vi "Add to Application MUXList.vi"(7 "Replace if found? (F)":bool, 8 "error in (no error)":errorcluster, 9 "Destinations":string[](array[string]), 10 "Source":string, 11 "SLSC Switch in":refnum<class "SLSC Switch.lvclass">) -> (0 "error out":errorcluster, 1 "New Entry?":bool, 3 "SLSC Switch out":refnum<class "SLSC Switch.lvclass">)   [LabVIEW 2016, in "SLSC Switch.lvlib" / "SLSC Switch.lvclass"]
uses:
  SLSC Switch.lvclass
  SLSC Switch.lvclass/SLSC Switch.ctl
  Controls/MuxList Entry.ctl
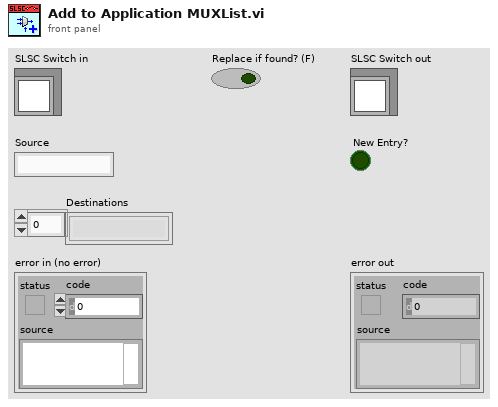
[diagram p1: front panel]
types:
  T1 = typedef "SLSC Switch.lvlib/SLSC Switch.lvclass/MuxList Entry.ctl" = cluster{"Source":string, "Destinations":string[]}
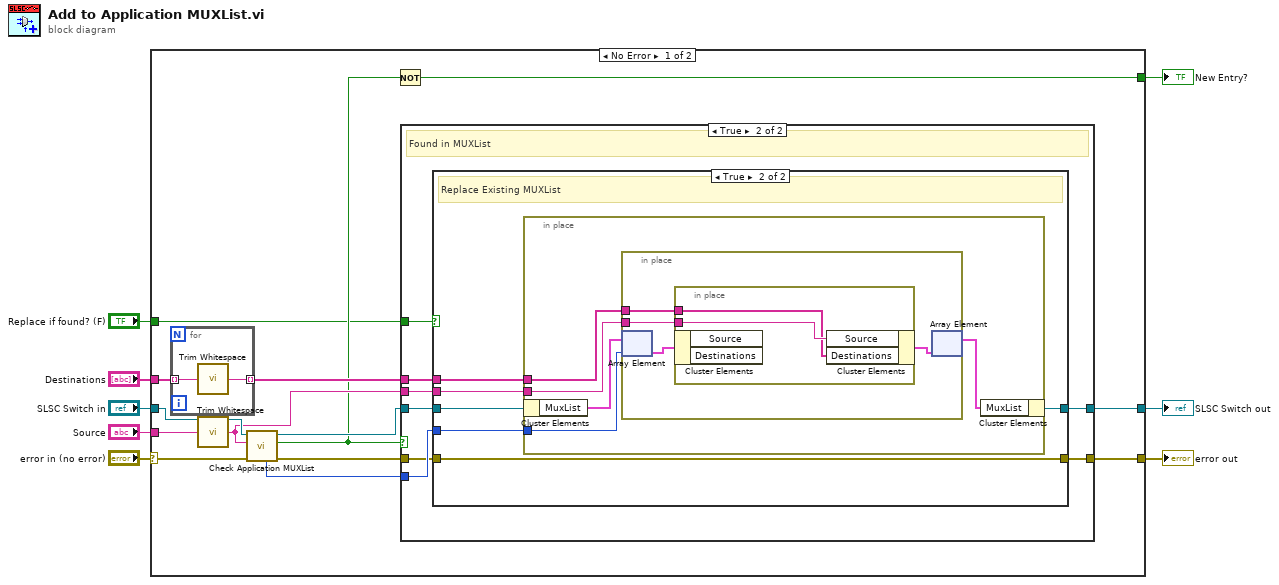
[diagram p0: block diagram]
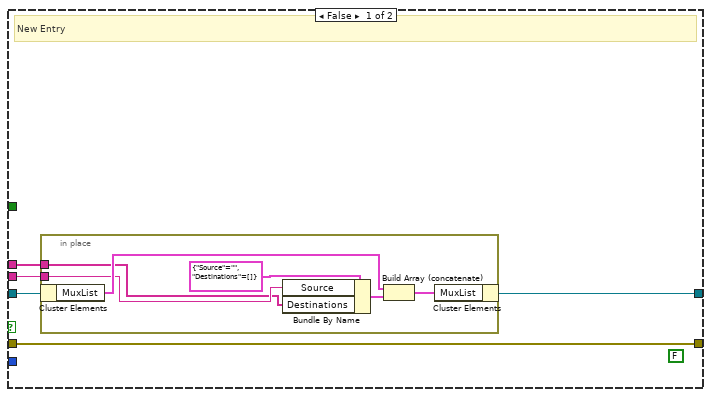
[diagram p2: hidden frame]
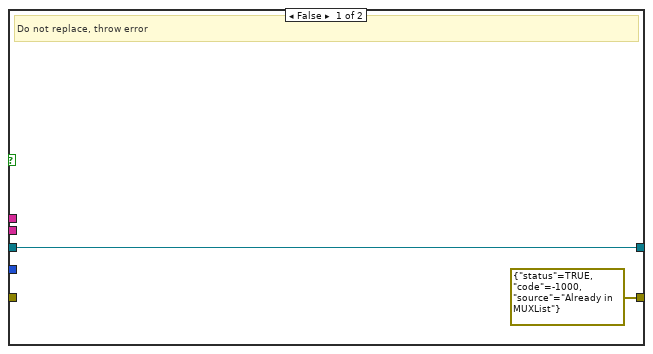
[diagram p3: hidden frame]
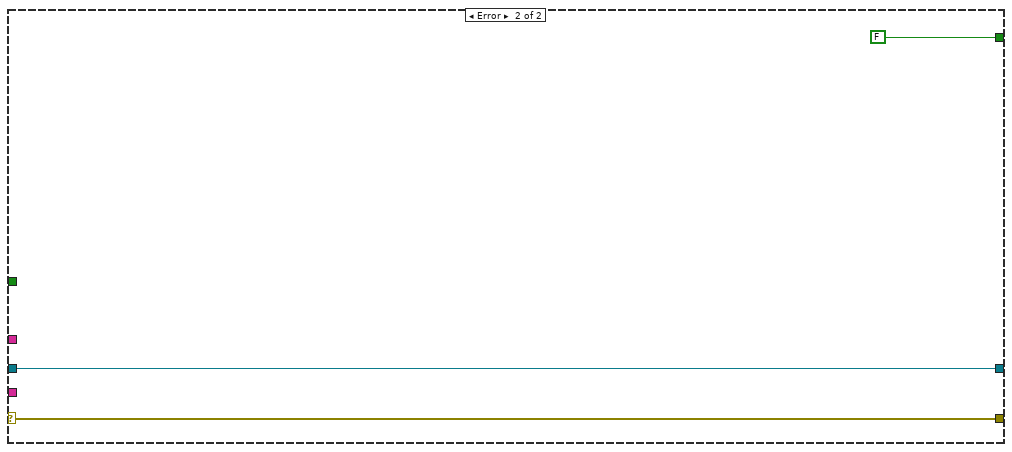
[diagram p4: hidden frame]
diagram:
  n1 = case shown="No Error" "error in (no error)" {
    selector: "error in (no error)" -> [w16 w65]
    tunnel: [w10 w65] -> w7
    tunnel: [w22 w64] -> w5
    tunnel: "SLSC Switch in" -> [w18 w64]
    tunnel: "Source" -> [w21 _]
    tunnel: [w14 FALSE] -> w3
    tunnel: "Destinations" -> [w20 _]
    tunnel: "Replace if found? (F)" -> [w11 _]
    frame No Error {
      n2 = for {
        tunnel: w20 -> [w24] mode=indexing
        tunnel: [w23] -> w19 mode=indexing
        n3 = call <vilib>:"Trim Whitespace.vi"("string"=w24) -> ("trimmed string"=w23:string)  [unwired: 1 in]
      }
      n4 = call <vilib>:"Trim Whitespace.vi"("string"=w21) -> ("trimmed string"=w15:string)  [unwired: 1 in]
      n5 = call "Check Application MUXList.vi"("error in (no error)"=w16, "Source"=w15, "SLSC Switch in"=w18) -> ("error out"=w9:errorcluster, "found?"=w13:bool, "SLSC Switch out"=w17:refnum<class "SLSC Switch.lvclass">, "index"=w12:i32)  [unwired: 4 in, 1 out]
      n6 = Not(x=w13) -> (.not. x?=w14:bool)
      n7 = case shown="True" w13 {
        tunnel: [w29 w38] -> w22
        tunnel: w17 -> [w28 w41]
        tunnel: w15 -> [w27 w40]
        tunnel: w19 -> [w26 w39]
        tunnel: w12 -> [_ w43]
        tunnel: w11 -> [_ w42]
        tunnel: [w25 w37] -> w10
        tunnel: w9 -> [w25 w36]
        frame False {
          (unwired) FALSE
          # "New Entry"
          n8 = in-place {
            in-place-border: w27 -> [w33]
            in-place-border: w26 -> [w32]
            n9 = in-place-cluster #1(w28) -> ("MuxList"=w35:T1[])
            n10 = Bundle By Name(cluster=T1 {"Source"="", "Destinations"=[]} ("Mux"), "Source"=w33, "Destinations"=w32) -> (w31:T1)
            n11 = Build Array (concatenate)(w35, w31) -> (w30:T1[])
            n12 = in-place-cluster #1("MuxList"=w30) -> (w29:refnum<class "SLSC Switch.lvclass">)
          }
        }
        frame True {
          # "Found in MUXList"
          n13 = case shown="True" w42 {
            tunnel: w43 -> [_ w50]
            tunnel: w41 -> [w45 w51]
            tunnel: w40 -> [_ w49]
            tunnel: w39 -> [_ w48]
            tunnel: [w45 w47] -> w38
            tunnel: [errorcluster {"status"=TRUE, "code"=-1000, "source"="Already in MUXList"} ("error out") w46] -> w37
            tunnel: w36 -> [_ w46]
            frame False {
              # "Do not replace, throw error"
            }
            frame True {
              # "Replace Existing MUXList"
              n14 = in-place {
                in-place-border: w50 -> [w55]
                in-place-border: w49 -> [w54]
                in-place-border: w48 -> [w53]
                n15 = in-place-cluster #2(w51) -> ("MuxList"=w56:T1[])
                n16 = in-place {
                  in-place-border: w54 -> [w59]
                  in-place-border: w53 -> [w58]
                  n17 = in-place-array #3(w56, w55) -> (w60:T1)
                  n18 = in-place {
                    in-place-border: w59 -> [w62]
                    in-place-border: w58 -> [w61]
                    n19 = in-place-cluster #4(w60) -> ()  [unwired: 2 out]
                    n20 = in-place-cluster #4("Source"=w62, "Destinations"=w61) -> (w57:T1)
                  }
                  n21 = in-place-array #3(w57) -> (w52:T1[])  [unwired: 1 out]
                }
                n22 = in-place-cluster #2("MuxList"=w52) -> (w47:refnum<class "SLSC Switch.lvclass">)
              }
            }
          }
        }
      }
    }
    frame Error {
    }
  }
  "error out" <- w7
  "SLSC Switch out" <- w5
  "New Entry?" <- w3
